vi "http check to keep listening.vi"(11 "application request in":T1) -> (2 "stop listening":bool, 3 "application request out":T1)   [LabVIEW 2016, in "Basic HTTP server.lvclass"]
uses:
  Basic HTTP server.lvclass
  http request.ctl
  http method.ctl
  http header data.ctl
  headers/http headers.lvlib
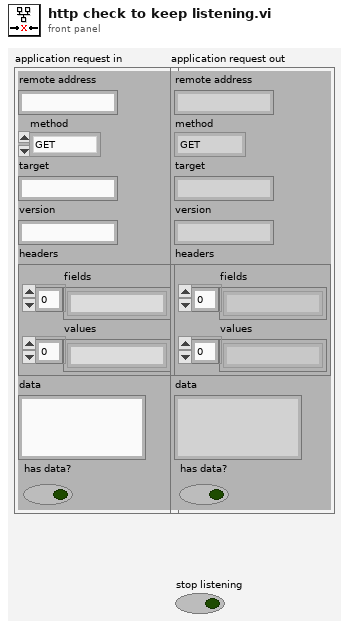
[diagram p1: front panel]
types:
  T1 = typedef "Basic HTTP server.lvclass/http request.ctl" = cluster{"remote address":string, "method":T2, "target":string, "version":string, "headers":T3, "data":string, "has data?":bool}
  T2 = typedef "Basic HTTP server.lvclass/http method.ctl" = enum16{"GET", "POST", "PUT", "DELETE", "HEAD", "OPTIONS", "upgrade"}
  T3 = typedef "http headers.lvlib/http header data.ctl" = cluster{"fields":string[], "values":string[]}
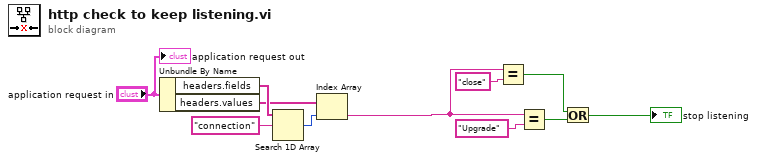
[diagram p0: block diagram]
diagram:
  n1 = Unbundle By Name("application request in") -> ("headers.fields"=w11:string[], "headers.values"=w8:string[])
  n2 = Search 1D Array(1D array=w11, element="connection" ("name")) -> (index of element=w9:i32)  [unwired: 1 in]
  n3 = Index Array(array=w8, index=w9) -> (element=w7:string)
  n4 = Equal?(x=w7, y="close" ("name")) -> (x = y?=w4:bool)
  n5 = Equal?(x=w7, y="Upgrade" ("name")) -> (x = y?=w1:bool)
  n6 = Or(x=w4, y=w1) -> (x .or. y?=→"stop listening":bool)
  "application request out" <- "application request in"
